vi "NI-DAQmx.vi"() -> (0 "error out":errorcluster)   [LabVIEW 2015]
uses:
  <vilib>/DAQmx/read.llb/DAQmx Read (Analog 2D DBL NChan NSamp).vi
  Globals/Meas_global.vi
  PWA/PWAtasksGLOBAL.vi
  <vilib>/DAQmx/miscellaneous.llb/DAQmx Fill In Error Info.vi
  <vilib>/DAQmx/configure/timing.llb/DAQmx Timing (Sample Clock).vi
  <vilib>/DAQmx/create/channels.llb/DAQmx Create Channel (AI-Voltage-Basic).vi
  <resource>/objmgr/daqmx.rc
panel:
  out "AuditTrail":string[](array[string])
  out "input terminal configuration":i32(ring)=10106 items=["default"=-1, "RSE"=10083, "NRSE"=10078, "Differential"=10106, "Pseudodifferential"=12529]
  out "AI.Voltage.Rngs":dbl[](array[numeric])=[-10.0, 10.0]
  out "TotalSampPerChanAcquired":dbl=1024.0
  out "AvailSampPerChan":u32
  out "CurrReadPos":dbl=1024.0
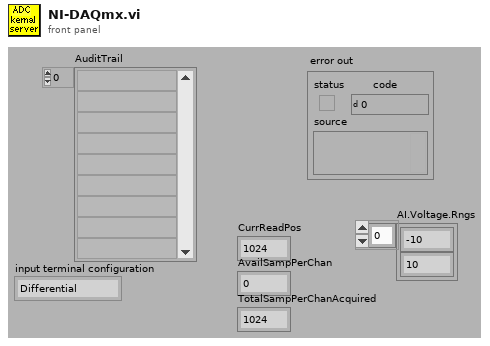
[diagram p1: front panel]
types:
  T1 = typedef "Ch_and_Spans.ctl" = cluster{"high limit (10V)":sgl, "low limit (-10V)":sgl, "Ch No":i16, "Var name":string, "Use Latest Calib":bool}
  T2 = typedef "LDA_Setup.ctl" = cluster{"dimensions":enum16{"1D", "2D"}, "Analogue Freq Multiplier":dbl}
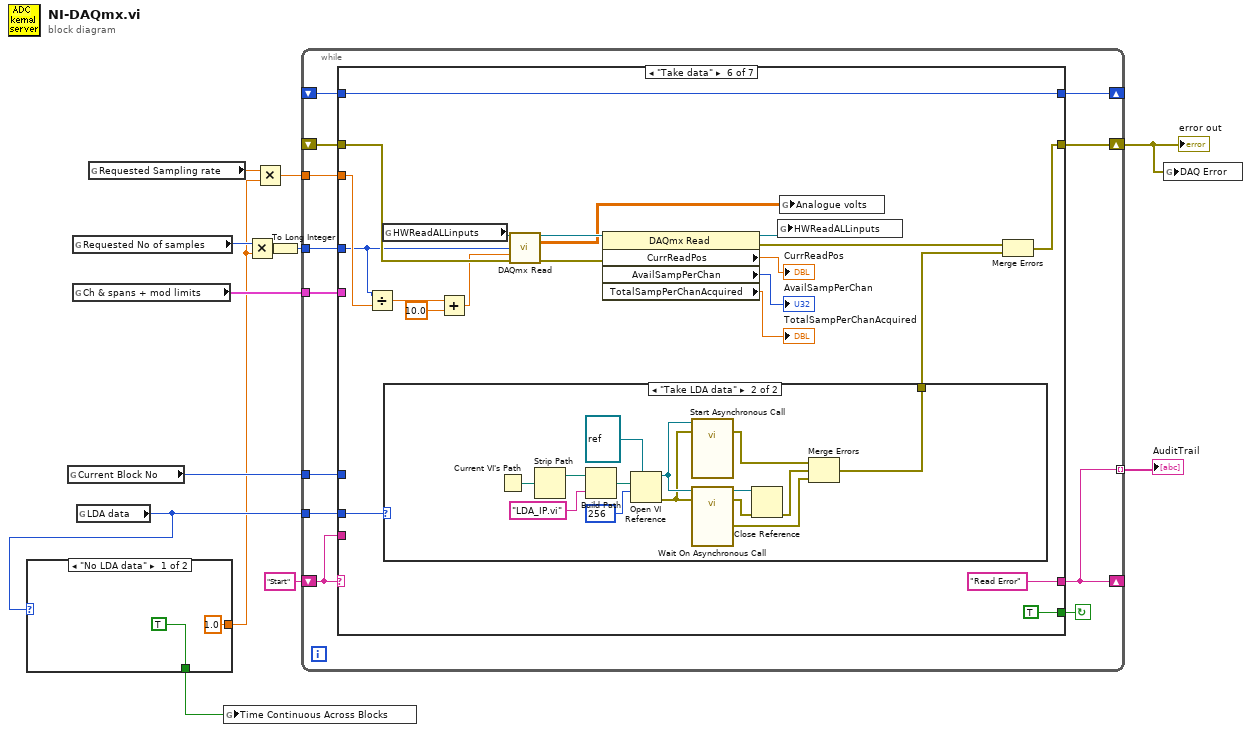
[diagram p0: block diagram]
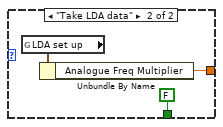
[diagram p2: hidden frame]
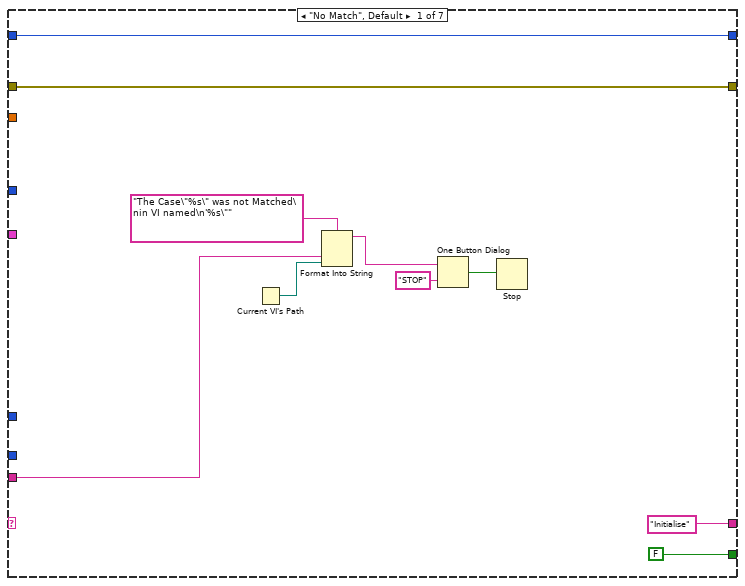
[diagram p3: hidden frame]
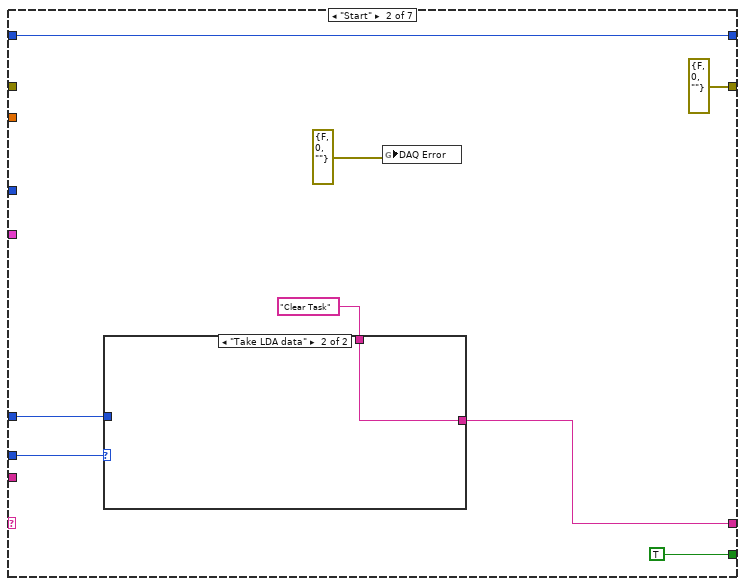
[diagram p4: hidden frame]
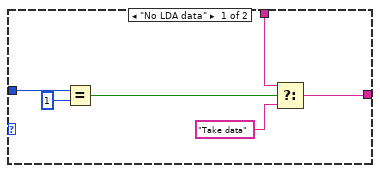
[diagram p5: hidden frame]
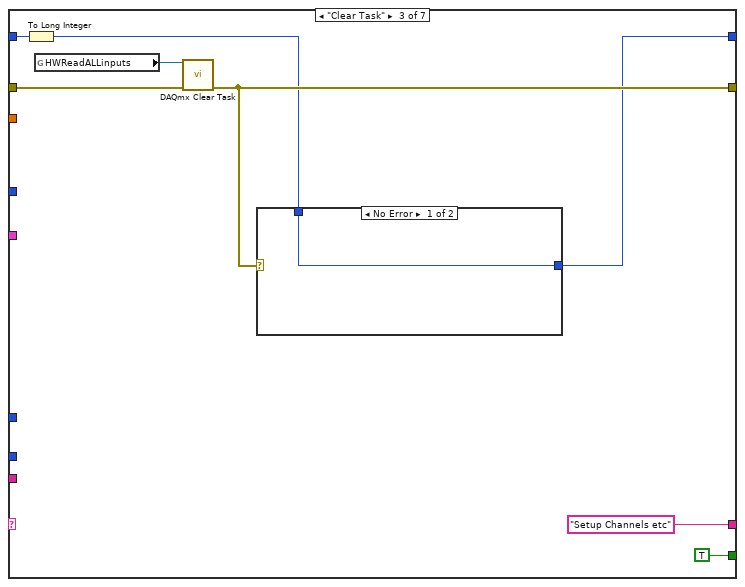
[diagram p6: hidden frame]
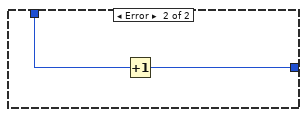
[diagram p7: hidden frame]
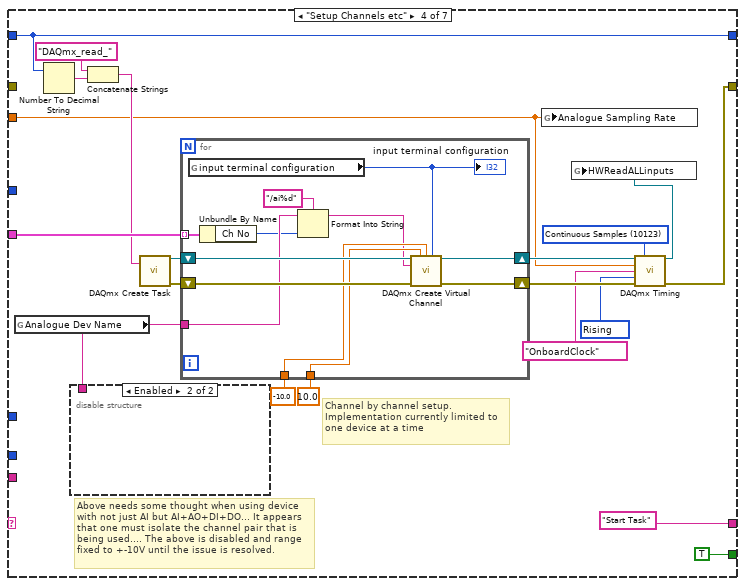
[diagram p8: hidden frame]
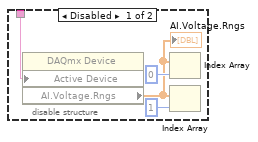
[diagram p9: hidden frame]
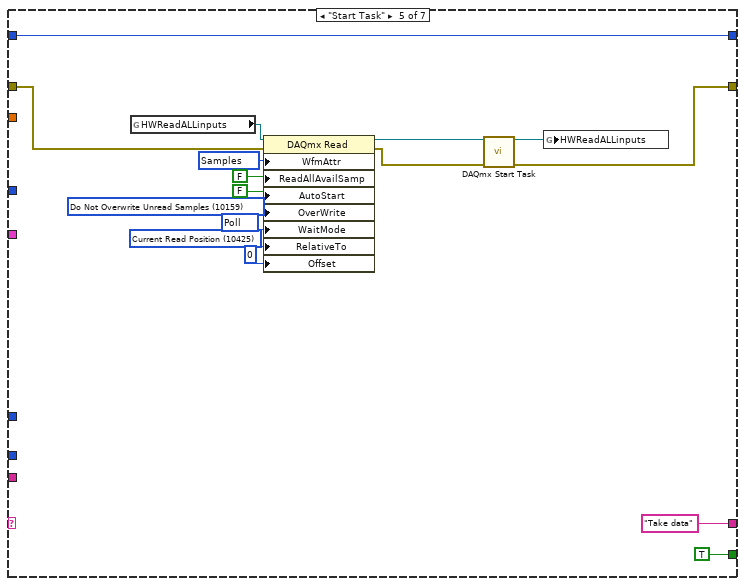
[diagram p10: hidden frame]
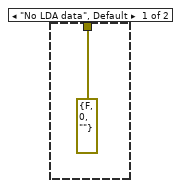
[diagram p11: hidden frame]
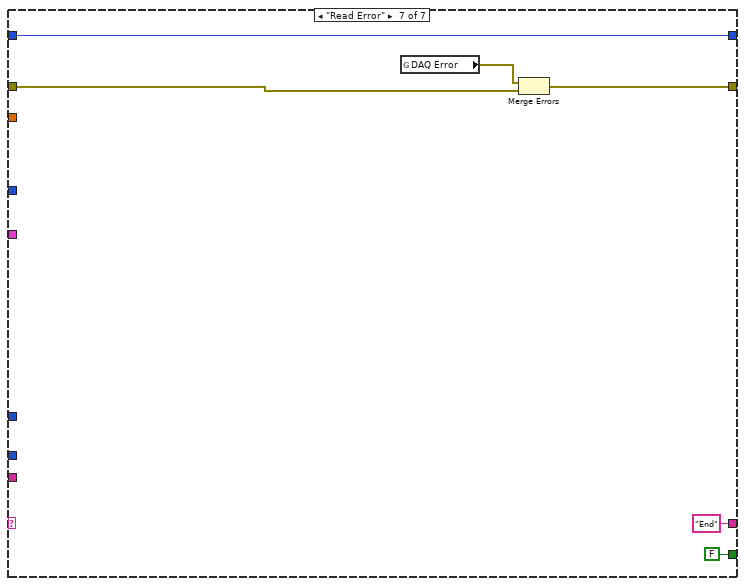
[diagram p12: hidden frame]
diagram:
  n1 = global read "Meas_global.vi" "Current Block No"() -> (w11:i32)
  n2 = global read "Meas_global.vi" "Requested No of samples"() -> (w7:i32)
  n3 = global read "Meas_global.vi" "Ch & spans + mod limits"() -> (w12:T1[])
  n4 = global read "Meas_global.vi" "LDA data"() -> (w9:enum16{"No LDA data", "Take LDA data"})
  n5 = case shown="\"No LDA data\"" w9 {
    tunnel: [1.0 ("Analogue Freq Multiplier") w17] -> w5
    tunnel: [TRUE ("Time Continuous across Blocks") FALSE ("Time Continuous across Blocks")] -> w1
    frame "No LDA data" {
    }
    frame "Take LDA data" {
      n6 = global read "Meas_global.vi" "LDA set up"() -> (w18:T2)
      n7 = Unbundle By Name(w18) -> ("Analogue Freq Multiplier"=w17:dbl)
    }
  }
  n8 = global read "Meas_global.vi" "Requested Sampling rate"() -> (w6:dbl)
  n9 = global write "Meas_global.vi" "Time Continuous Across Blocks"(w1) -> ()
  n10 = Multiply(x=w7, y=w5) -> (x*y=w8:dbl)
  n11 = Multiply(x=w6, y=w5) -> (x*y=w4:dbl)
  n12 = To Long Integer(number=w8) -> (32bit integer=w3:i32)
  n13 = while {
    shift-left: "Start" -> [w29]
    shift-right: [w19] -> _
    shift-right: [w23] -> w10
    shift-left: _ -> [w28]
    tunnel: w4 -> [w27]
    tunnel: w3 -> [w26]
    tunnel: w11 -> [w25]
    tunnel: w12 -> [w24]
    shift-right: [w22] -> _
    shift-left: _ -> [w21]
    tunnel: w9 -> [w20]
    tunnel: [w19] -> w2 mode=indexing
    stop <- w30 continue-if-true
    n14 = case shown="\"Take data\"" w29 {
      tunnel: [FALSE TRUE TRUE TRUE TRUE TRUE FALSE] -> w30
      tunnel: ["Initialise" w46 "Setup Channels etc" "Start Task" "Take data" "Read Error" "End" ("f")] -> w19
      tunnel: w29 -> [w35 _ _ _ _ _ _]
      tunnel: [w32 errorcluster {"status"=FALSE, "code"=0, "source"=""} ("error out") w59 w80 w104 w120 w158] -> w23
      tunnel: w28 -> [w32 _ w60 _ w109 w139 w159]
      tunnel: w27 -> [_ _ _ w69 _ w128 _]
      tunnel: w26 -> [_ _ _ _ _ w119 _]
      tunnel: w25 -> [_ w43 _ _ _ _ _]
      tunnel: w24 -> [_ _ _ w79 _ _ _]
      tunnel: [w31 w45 w58 w68 w107 w129 w157] -> w22
      tunnel: w21 -> [w31 w45 w57 w68 w107 w129 w157]
      tunnel: w20 -> [_ w42 _ _ _ w123 _]
      frame "No Match", Default {
        n15 = Current VI's Path() -> (path=w34:path)
        n16 = Format Into String(format string="The Case\"%s\" was not Matched\nin VI named\n'%s\"" ("Format String"), w35, w34) -> (resulting string=w38:string)  [unwired: 2 in, 1 out]
        n17 = One Button Dialog(message=w38, button name ("OK")="STOP") -> (true=w36:bool)
        n18 = Stop(stop? (T)=w36) -> ()
      }
      frame "Start" {
        n19 = case shown="\"Take LDA data\"" w42 {
          tunnel: "Clear Task" -> [w54 w55]
          tunnel: [w52 w55] -> w46
          tunnel: w43 -> [w51 _]
          frame "No LDA data" {
            n20 = Equal?(x=w51, y=1) -> (x = y?=w49:bool)
            n21 = Select(t=w54, s=w49, f="Take data") -> (s? t:f=w52:string)
          }
          frame "Take LDA data" {
          }
        }
        n22 = global write "Meas_global.vi" "DAQ Error"(errorcluster {"status"=FALSE, "code"=0, "source"=""} ("DAQ Error")) -> ()
      }
      frame "Clear Task" {
        n23 = To Long Integer(number=w57) -> (32bit integer=w56:i32)
        n24 = global read "PWAtasksGLOBAL.vi" "HWReadALLinputs"() -> (w61:refnum<k21>)
        n25 = call <vilib>:"DAQmx Clear Task.vi"("task in"=w61, "error in"=w60) -> ("error out"=w59:errorcluster)  [unwired: 13 out]
        n26 = case shown="No Error" w59 {
          tunnel: [w64 w65] -> w58
          tunnel: w56 -> [w64 w66]
          frame No Error {
          }
          frame Error {
            n27 = Increment(x=w66) -> (x+1=w65:i32)
          }
        }
      }
      frame "Setup Channels etc" {
        w77 = 10280 items=["Rising"=10280, "Falling"=10171] ("active edge")
        w83 = 10123 items=["Finite Samples"=10178, "Continuous Samples"=10123, "Hardware Timed Single Point"=12522] ("sample mode")
        # "Above needs some thought when using device with not just AI but AI+AO+DI+DO... It appears that one must isolate the channel pair that is being used.... The above is disabled and range fixed to +-10V until the issue is resolved."
        # "Channel by channel setup. Implementation currently limited to one device at a time"
        n28 = global read "PWAtasksGLOBAL.vi" "Analogue Dev Name"() -> (w72:string)
        n29 = Number To Decimal String(number=w68) -> (decimal integer string=w67:string)  [unwired: 1 in]
        n30 = disable-structure shown="Enabled" {
          disable-tunnel: w72 -> [w87 _]
          frame Disabled {
            n31 = property class="DAQmx Device"("Active Device"=w87) -> ("AI.Voltage.Rngs"=w88:dbl[])  [unwired: 2 in, 2 out]
            "AI.Voltage.Rngs" <- w88
            n32 = Index Array(array=w88, index=0) -> ()  [unwired: 1 out]
            n33 = Index Array(array=w88, index=1) -> ()  [unwired: 1 out]
          }
          frame Enabled {
          }
        }
        n34 = Concatenate Strings("DAQmx_read_" ("new task name"), w67) -> (w70:string)
        n35 = call <vilib>:"DAQmx Create Task.vi"("new task name"=w70) -> ("task out"=w81:refnum<k21>, "error out"=w84:errorcluster)  [unwired: 4 in, 9 out]
        n36 = for {
          tunnel: w79 -> [w102] mode=indexing
          shift-right: [w100] -> w82
          shift-left: w81 -> [w101]
          shift-right: [w98] -> w85
          shift-left: w84 -> [w99]
          tunnel: w72 -> [w95]
          tunnel: -10.0 -> [w97]
          tunnel: 10.0 -> [w96]
          n37 = global read "Meas_global.vi" "input terminal configuration"() -> (w91:i32)
          "input terminal configuration" <- w91
          n38 = Unbundle By Name(w102) -> ("Ch No"=w94:i16)
          n39 = Format Into String(format string="/ai%d", initial string=w95, w94) -> (resulting string=w92:string)  [unwired: 1 in, 1 out]
          n40 = call-poly <vilib>:"DAQmx Create Virtual Channel.vi"("task in"=w101, "maximum value"=w96, "minimum value"=w97, "input terminal configuration"=w91, "physical channels"=w92, "error in"=w99) -> ("task out"=w100:refnum<k21>, "error out"=w98:errorcluster)  [unwired: 3 in, 5 out]
        }
        n41 = global write "Meas_global.vi" "Analogue Sampling Rate"(w69) -> ()
        n42 = call-poly <vilib>:"DAQmx Timing.vi"("task/channels in"=w82, "sample mode"=w83, "rate"=w69, "source"=tag "OnboardClock", "active edge"=w77, "error in"=w85) -> ("task out"=w78:refnum<k21>, "error out"=w80:errorcluster)  [unwired: 1 in, 7 out]
        n43 = global write "PWAtasksGLOBAL.vi" "HWReadALLinputs"(w78) -> ()
      }
      frame "Start Task" {
        w112 = 10425 items=["First Sample"=10424, "Current Read Position"=10425, "Reference Trigger"=10426, "First Pretrigger Sample"=10427, "Most Recent Sample"=10428] ("RelativeTo")
        w113 = 12524 items=["Wait For Interrupt"=12523, "Poll"=12524, "Yield"=12525, "Sleep"=12547] ("WaitMode")
        w114 = 10159 items=["Overwrite Unread Samples"=10252, "Do Not Overwrite Unread Samples"=10159] ("OverWrite")
        w116 = 10287 items=["Samples"=10287, "Samples and Timing"=10140, "Samples, Timing, and Attributes"=10141] ("WfmAttr")
        n44 = global read "PWAtasksGLOBAL.vi" "HWReadALLinputs"() -> (w110:refnum<k21>)
        n45 = property class="DAQmx Read"(reference=w110, error in=w109, "WfmAttr"=w116, "ReadAllAvailSamp"=FALSE, "AutoStart"=FALSE, "OverWrite"=w114, "WaitMode"=w113, "RelativeTo"=w112, "Offset"=0) -> (reference out=w105:refnum<k21>, error out=w106:errorcluster)
        n46 = call <vilib>:"DAQmx Start Task.vi"("task/channels in"=w105, "error in"=w106) -> ("task out"=w103:refnum<k21>, "error out"=w104:errorcluster)  [unwired: 12 out]
        n47 = global write "PWAtasksGLOBAL.vi" "HWReadALLinputs"(w103) -> ()
      }
      frame "Take data" {
        n48 = Divide(x=w119, y=w128) -> (x/y=w127:dbl)
        n49 = global read "PWAtasksGLOBAL.vi" "HWReadALLinputs"() -> (w132:refnum<k21>)
        n50 = case shown="\"Take LDA data\"" w123 {
          tunnel: [errorcluster {"status"=FALSE, "code"=0, "source"=""} ("error out") w141] -> w122
          frame "No LDA data", Default {
          }
          frame "Take LDA data" {
            n51 = Current VI's Path() -> (path=w152:path)
            n52 = Strip Path(path=w152) -> (stripped path=w151:path)  [unwired: 1 out]
            n53 = Build Path(base path=w151, name or relative path="LDA_IP.vi") -> (appended path=w153:path)
            n54 = Open VI Reference(type specifier VI Refnum (for type only)=refnum<vi> refnum, vi path=w153, options=256) -> (vi reference=w148:refnum<vi>, error out=w147:errorcluster)  [unwired: 3 in]
            n55 = call-by-ref "Start Asynchronous Call"(reference=w148, error in=w147) -> (error out=w144:errorcluster)  [unwired: 1 in, 2 out]
            n56 = call-by-ref "Wait On Asynchronous Call"(reference=w148, error in=w147) -> (reference out=w146:refnum<vi>, error out=w145:errorcluster, 0:"error out"=w142:errorcluster)  [unwired: 1 in]
            n57 = Close Reference(reference=w146, error in (no error)=w145) -> (error out=w143:errorcluster)
            n58 = Merge Errors(w144, w143, w142) -> (w141:errorcluster)
          }
        }
        n59 = Add(x=w127, y=10.0) -> (x+y=w125:dbl)
        n60 = call-poly <vilib>:"DAQmx Read.vi"("task/channels in"=w132, "number of samples per channel"=w119, "timeout"=w125, "error in"=w139) -> ("task out"=w136:refnum<k21>, "data"=w124:dbl[][], "error out"=w131:errorcluster)  [unwired: 9 out]
        n61 = property class="DAQmx Read"(reference=w136, error in=w131) -> (reference out=w135:refnum<k21>, error out=w121:errorcluster, "CurrReadPos"=→"CurrReadPos":dbl, "AvailSampPerChan"=→"AvailSampPerChan":u32, "TotalSampPerChanAcquired"=→"TotalSampPerChanAcquired":dbl)
        n62 = global write "PWAtasksGLOBAL.vi" "HWReadALLinputs"(w135) -> ()
        n63 = global write "Meas_global.vi" "Analogue volts"(w124) -> ()
        n64 = Merge Errors(w121, w122) -> (w120:errorcluster)
      }
      frame "Read Error" {
        n65 = global read "Meas_global.vi" "DAQ Error"() -> (w160:errorcluster)
        n66 = Merge Errors(w160, w159) -> (w158:errorcluster)
      }
    }
  }
  "error out" <- w10
  "AuditTrail" <- w2
  n67 = global write "Meas_global.vi" "DAQ Error"(w10) -> ()
